vi "Build version to string.vi"(11 "Build Version":T1) -> (2 "Build Version (String)":string)   [LabVIEW 2021, in "App-Builder Library.lvlib" / "Builder.lvclass"]
uses:
  Builder.lvclass
  <vilib>/Utility/error.llb/whitespace.ctl
  <vilib>/AppBuilder/AB_API_Simple/Build Specification Version.ctl
  <vilib>/AppBuilder/AB_API_Simple/NI_App_Builder_API.lvlib
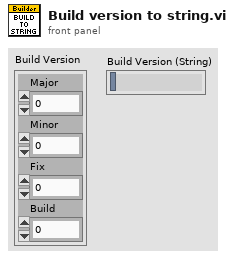
[diagram p1: front panel]
types:
  T1 = typedef "NI_App_Builder_API.lvlib/Build Specification Version.ctl" = cluster{"Major":u16, "Minor":u16, "Fix":u16, "Build":u16}
  T2 = typedef "whitespace.ctl" = u16
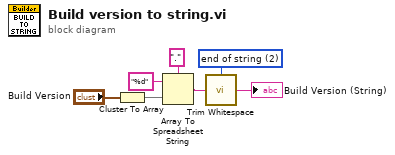
[diagram p0: block diagram]
diagram:
  w1 = T2 2 items=["both", "start of string", "end of string"] ("location (both)")
  n1 = Cluster To Array(cluster="Build Version") -> (array=w6:u16[])
  n2 = Array To Spreadsheet String(delimiter (Tab)=".", array=w6, 3:"%d" ("format string")) -> (spreadsheet string=w3:string)
  n3 = call <vilib>:"Trim Whitespace.vi"("string"=w3, "location (both)"=w1) -> ("trimmed string"=→"Build Version (String)":string)
